vi "11100 UI.vi"(8 "error in (no error)":errorcluster, 11 "Node Ptr":T1 format="%.0x") -> (0 "error out":errorcluster)   [LabVIEW 2017, in "Modules.lvlib" / "11100.lvclass"]
uses:
  11100.lvclass
  <vilib>/NI Veristand/Custom Device API/Custom Device Item Ref.ctl
  RSI Module/SubPanel Command.ctl
  C:/Users/dbuck/Documents/GitHub/Scan-Engine-Custom-Device-Classes/Source/RemIO Module/RemIO Module.lvclass
  11100.lvclass/11100.ctl
  <vilib>/indcomecat/Remote IO/typedefs/REM-11102/channul number REM-11102.ctl
  RemIO Module/RemIO Module.lvclass
  <vilib>/indcomecat/Remote IO/NI ECAT Remote IO.lvlib
  <vilib>/NI Veristand/Custom Device API/Custom Device API.lvlib
  RSI Module/RSI Module.lvclass
panel:
  in  "Output Range":u8[](array[ring])=[0, 0, 0, 0] items=["0 V ... 10 V"=0, "-10 V ... 10 V"=1, "0 V ... 5 V"=2, "-5 V ... 5V"=3, "0 mA ... 20 mA"=4, "4 mA ... 20 mA"=6, "Channel inactive"=15]
  in  "Mean Value":u8[](array[ring])=[1, 1, 1, 1] items=["no mean-value"=1, "4-sample"=2, "16-sample"=0, "32-sample"=3]
  in  "Input Filter Time":u8[](array[ring])=[0, 0, 0, 0] items=["30 Hz", "12 kHz"]
  out "_MeanVallabel":string="Mean-Value"
  out "_InFilterlabel":string="Input Filter Time"
  out "_Chan0Label":string="Channel 0"
  out "_Chan1Label":string="Channel 1"
  out "_Chan2Label":string="Channel 2"
  out "_Chan3Label":string="Channel 3"
  out "_Rangelabel":string="Measuring Range"
  in  "SubPanel Event":refnum<user-event>
  in  "Header":cluster{"Section Name":string}={"Section Name"="NI REM-11100 Settings"}
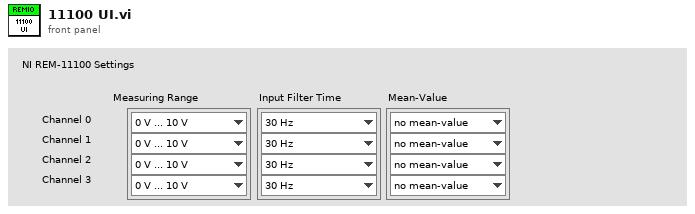
[diagram p1: front panel]
types:
  T1 = typedef "Custom Device API.lvlib/Custom Device Item Ref.ctl" = u64
  T2 = typedef "NI ECAT Remote IO.lvlib/channel number REM-11100.ctl" = u8
  T3 = typedef "NI ECAT Remote IO.lvlib/input filter time REM-11100.ctl" = u8
  T4 = typedef "NI ECAT Remote IO.lvlib/mean-value REM-11100.ctl" = u8
  T5 = typedef "NI ECAT Remote IO.lvlib/measuring range REM-11100.ctl" = u8
  T6 = cluster{"channel number":T2, "input filter time":T3, "mean-value":T4, "measuring range":T5}[]
  T7 = typedef "Modules.lvlib/RSI Module.lvclass/SubPanel Command.ctl" = enum16{"Stop"}
  T8 = typedef "NI ECAT Remote IO.lvlib/channul number REM-11102.ctl" = u8
  T9 = cluster{"channel number":T8, "Input Filter 3":u8, "Mean Value 3":u8, "Output Range 3":u8}
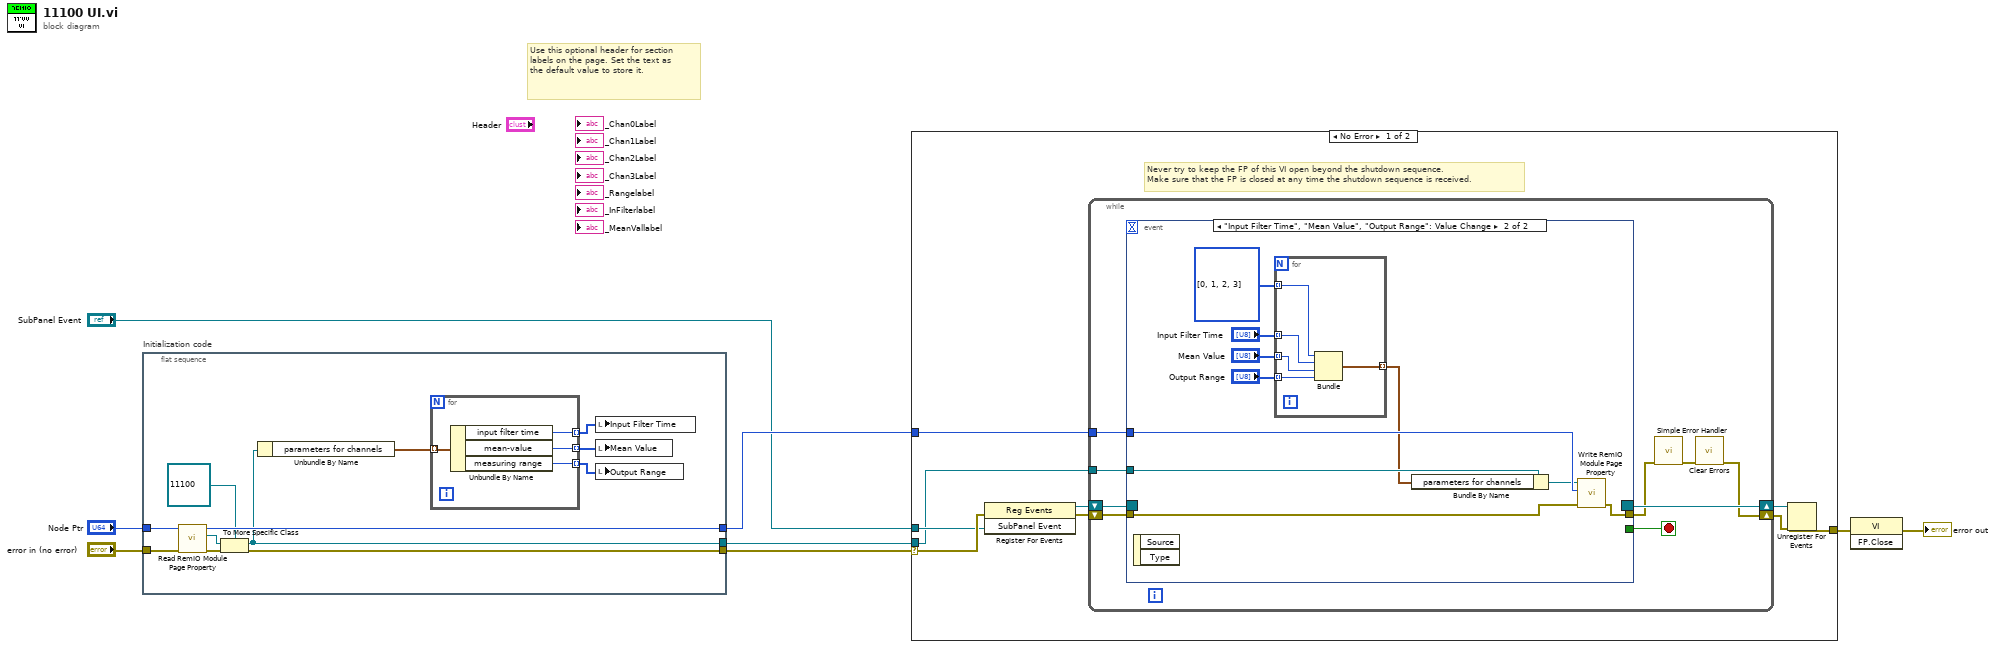
[diagram p0: block diagram]
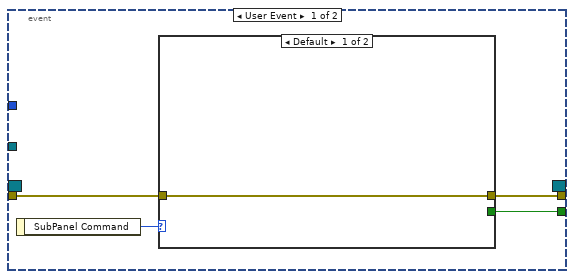
[diagram p2: hidden frame]
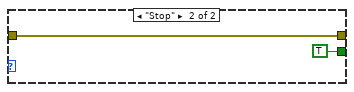
[diagram p3: hidden frame]
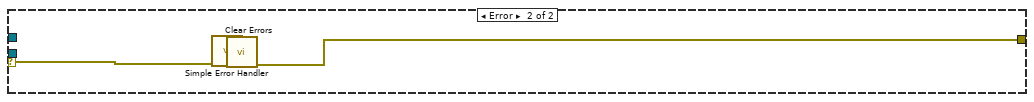
[diagram p4: hidden frame]
diagram:
  # "Use this optional header for section labels on the page. Set the text as the default value to store it."
  n1 = flat-sequence "Initialization code" {
    tunnel: "error in (no error)" -> [w19]
    tunnel: "Node Ptr" -> [w20]
    tunnel: [w15] -> w2
    tunnel: [w18] -> w5
    tunnel: [w14] -> w1
    frame #0 {
      n2 = call "Read RemIO Module Page Property.vi"("error in (no error)"=w19, "Node Ptr In"=w20) -> ("error out"=w17:errorcluster, "RemIO Module"=w16:refnum<class "RemIO Module.lvclass">, "Node Ptr Out"=w18:T1)  [unwired: 7 in]
      n3 = To More Specific Class(target class=refnum<class "11100.lvclass"> refnum ("Modules.lvlib:11100.lvclass"), reference=w16, error in=w17) -> (specific class reference=w14:refnum<class "11100.lvclass">, error out=w15:errorcluster)
      n4 = Unbundle By Name(w14) -> ("parameters for channels"=w12:T6)
      n5 = for {
        tunnel: w12 -> [w24] mode=indexing
        tunnel: [w23] -> w10 mode=indexing
        tunnel: [w22] -> w11 mode=indexing
        tunnel: [w21] -> w9 mode=indexing
        n6 = Unbundle By Name(w24) -> ("input filter time"=w23:T3, "mean-value"=w22:T4, "measuring range"=w21:T5)
      }
      n7 = local write "Input Filter Time"(w10) -> ()
      n8 = local write "Mean Value"(w11) -> ()
      n9 = local write "Output Range"(w9) -> ()
    }
  }
  n10 = case shown="No Error" w2 {
    selector: w2 -> [w27 w67]
    tunnel: [w31 w65] -> w8
    tunnel: w5 -> [w28 _]
    tunnel: "SubPanel Event" -> [w26 _]
    tunnel: w1 -> [w25 _]
    frame No Error {
      # "Never try to keep the FP of this VI open beyond the shutdown sequence.\nMake sure that the FP is closed at any time the shutdown sequence is received."
      n11 = register-events(error in=w27, w26) -> (reference out=w29:refnum<event-registration>, error out=w30:errorcluster)  [unwired: 1 in]
      n12 = while {
        tunnel: w28 -> [w38]
        shift-right: [w35] -> w32
        shift-left: w30 -> [w41]
        shift-right: [w42] -> w33
        shift-left: w29 -> [w40]
        tunnel: w25 -> [w34]
        stop <- w39 stop-if-true
        n13 = event shown="[1] \"Input Filter Time\", \"Mean Value\", \"Output Range\": Value Change" {
          selector: w40 -> [_ _]
          dyn-events: [_ _] -> w42
          timeout: _ -> [_ _]
          tunnel: w41 -> [w45 w57]
          tunnel: [w43 _] -> w39
          tunnel: [w44 w56] -> w37
          tunnel: w38 -> [_ w58]
          tunnel: w34 -> [_ w59]
          event User Event {
            n14 = event-data() -> ("SubPanel Command"=w46:T7)  [unwired: 1 out]
            n15 = case shown="Default" w46 {
              tunnel: w45 -> [w47 w48]
              tunnel: [w47 w48] -> w44
              tunnel: [_ TRUE] -> w43
              frame Default {
              }
              frame "Stop" {
              }
            }
          }
          event "Input Filter Time", "Mean Value", "Output Range": Value Change {
            w51 = T8[] [0, 1, 2, 3] items=["AI0", "AI1", "AI2", "AI3"]
            n16 = event-data() -> ()  [unwired: 3 out]
            n17 = for {
              tunnel: "Output Range" -> [w64] mode=indexing
              tunnel: "Mean Value" -> [w63] mode=indexing
              tunnel: "Input Filter Time" -> [w61] mode=indexing
              tunnel: w51 -> [w62] mode=indexing
              tunnel: [w60] -> w50 mode=indexing
              n18 = Bundle("channel number"=w62, "Input Filter 3"=w61, "Mean Value 3"=w63, "Output Range 3"=w64) -> (w60:T9)  [unwired: 1 in]
            }
            n19 = Bundle By Name(cluster=w59, "parameters for channels"=w50) -> (w55:refnum<class "11100.lvclass">)
            n20 = call "Write RemIO Module Page Property.vi"("error in (no error)"=w57, "Node Ptr In"=w58, "RemIO Module"=w55) -> ("error out"=w56:errorcluster)  [unwired: 6 in, 2 out]
          }
        }
        n21 = call <vilib>:"Simple Error Handler.vi"("error in (no error)"=w37) -> ("error out"=w36:errorcluster)  [unwired: 1 in, 7 out]
        n22 = call <vilib>:"Clear Errors.vi"("error in (no error)"=w36) -> ("error out"=w35:errorcluster)  [unwired: 1 in, 5 out]
      }
      n23 = Unregister For Events(event registration refnum=w33, error in=w32) -> (error out=w31:errorcluster)
    }
    frame Error {
      n24 = call <vilib>:"Simple Error Handler.vi"("error in (no error)"=w67) -> ("error out"=w66:errorcluster)  [unwired: 1 in, 7 out]
      n25 = call <vilib>:"Clear Errors.vi"("error in (no error)"=w66) -> ("error out"=w65:errorcluster)  [unwired: 1 in, 5 out]
    }
  }
  n26 = invoke class="VI" method="FP.Close"(error in=w8) -> (error out=→"error out":errorcluster)  [unwired: 2 in, 2 out]
